vi "ModbusMaster.vi"(11 "queue in":refnum<queue>) -> ()   [LabVIEW 2014]
uses:
  controls/UI Data.ctl
  Project/Software/MyRIO Testing Software/Modbus.ctl
  <vilib>/Modbus/subvis/Modbus API/Modbus API.lvclass/Modbus API.ctl
  <vilib>/Modbus/subvis/Transmission Data Unit (ADU)/Transmission Data Unit/Transmission Data Unit.lvclass/Transmission Data Unit.ctl
  controls/Control ConfigurationSam.ctl
  <vilib>/Modbus/master/Modbus Master.lvclass
  <vilib>/Modbus/master/Data Access/Read Timeout/Set Read Timeout.vi
  <vilib>/Modbus/master/Data Access/Write Timeout/Set Write Timeout.vi
  <vilib>/Modbus/subvis/Modbus API/Read Transmission Data Unit.vi
  <vilib>/Modbus/subvis/Modbus API/Write Transmission Data Unit.vi
  <vilib>/Modbus/subvis/Transmission Data Unit (ADU)/Transmission Data Unit/Data Access/timeouts/Write read operation timeout.vi
  <vilib>/Modbus/subvis/Transmission Data Unit (ADU)/Transmission Data Unit/Data Access/timeouts/Write write operation timeout.vi
  <vilib>/Modbus/master/Data Access/Unit ID/Set Unit ID Property.vi
  <vilib>/Modbus/subvis/Transmission Data Unit (ADU)/Transmission Data Unit/Data Access/Unit ID/Write Unit ID.vi
  <vilib>/Modbus/master/Create Master Instance (Serial).vi
  <vilib>/Modbus/subvis/Transmission Data Unit (ADU)/Transmission Data Unit/Transmission Data Unit.lvclass
panel:
  out "PSoC PID Value":dbl
  out "Kp5":dbl=4.0
  out "Ki5":dbl=0.001
  out "Kd5":dbl
  in  "PIDScaler5":dbl=1000.0
  out "X":dbl
  out "Actual Values Written5":u16[](array[numeric])
  out "LabVIEW Heading":dbl
  out "Y":dbl
  out "PSoC Heading":dbl
  out "Values Read5":u16[](array[numeric])
  out "Values Read2":u16[](array[numeric])
  out "PositionLow2":u16
  out "PositionHigh2":i16
  out "SpeedRPS2":dbl
  out "SpeedRPM2":i16
  out "Motor Current2":dbl
  out "Position Full2":i32
  out "Setpoint Speed2":i16
  out "Actual Values Written2":u16[](array[numeric])
  out "Kd2":dbl
  out "Ki2":dbl=0.001
  out "Kp2":dbl=4.0
  in  "PIDScaler2":dbl=1000.0
  out "Values Read1":u16[](array[numeric])
  out "PositionLow1":u16
  out "PositionHigh1":i16
  out "SpeedRPS1":dbl
  out "SpeedRPM1":i16
  out "Motor Current1":dbl
  out "Position Full1":i32
  out "Setpoint Speed1":i16
  out "Actual Values Written1":u16[](array[numeric])
  out "Kd1":dbl
  out "Ki1":dbl=0.001
  out "Kp1":dbl=4.0
  in  "PIDScaler1":dbl=1000.0
  out "Setpoint Speed3":i16
  out "Actual Values Written3":u16[](array[numeric])
  out "Kd3":dbl
  out "Ki3":dbl=0.001
  out "Kp3":dbl=4.0
  in  "PIDScaler3":dbl=1000.0
  out "Values Read3":u16[](array[numeric])
  out "PositionLow3":u16
  out "PositionHigh3":i16
  out "SpeedRPS3":dbl
  out "SpeedRPM3":i16
  out "Motor Current3":dbl
  out "Position Full3":i32
  in  "PIDScaler4":dbl=1000.0
  out "Kp4":dbl=4.0
  out "Ki4":dbl=0.001
  out "Kd4":dbl
  out "Actual Values Written4":u16[](array[numeric])
  out "Setpoint Speed4":i16
  out "Position Full4":i32
  out "Motor Current4":dbl
  out "SpeedRPM4":i16
  out "SpeedRPS4":dbl
  out "PositionHigh4":i16
  out "PositionLow4":u16
  out "Values Read4":u16[](array[numeric])
  in  "Coil Values to Write":bool[](array[boolean])
  in  "Read Count 2":u16=10
  out "Coil Values Read":bool[](array[boolean])
  in  "flow control":u16(ring) items=["None", "XON/XOFF", "RTS/CTS", "XON/XOFF & RTS/CTS", "DTR/DSR", "XON/XOFF & DTR/DSR"]
  in  "parity":u16(ring) items=["None", "Odd", "Even"]
  in  "StartingSlave ID":u8=4
  in  "serial type":enum16{"RTU", "ASCII"}(ring)
  in  "VISA resource name":refnum<visa-resource-name>="ASRL3::INSTR"
  in  "baud rate":u32=115200
  # "Modbus Controller"
  # "Motor 1"
  # "Motor 2"
  # "Motor 3"
  # "Motor 4"
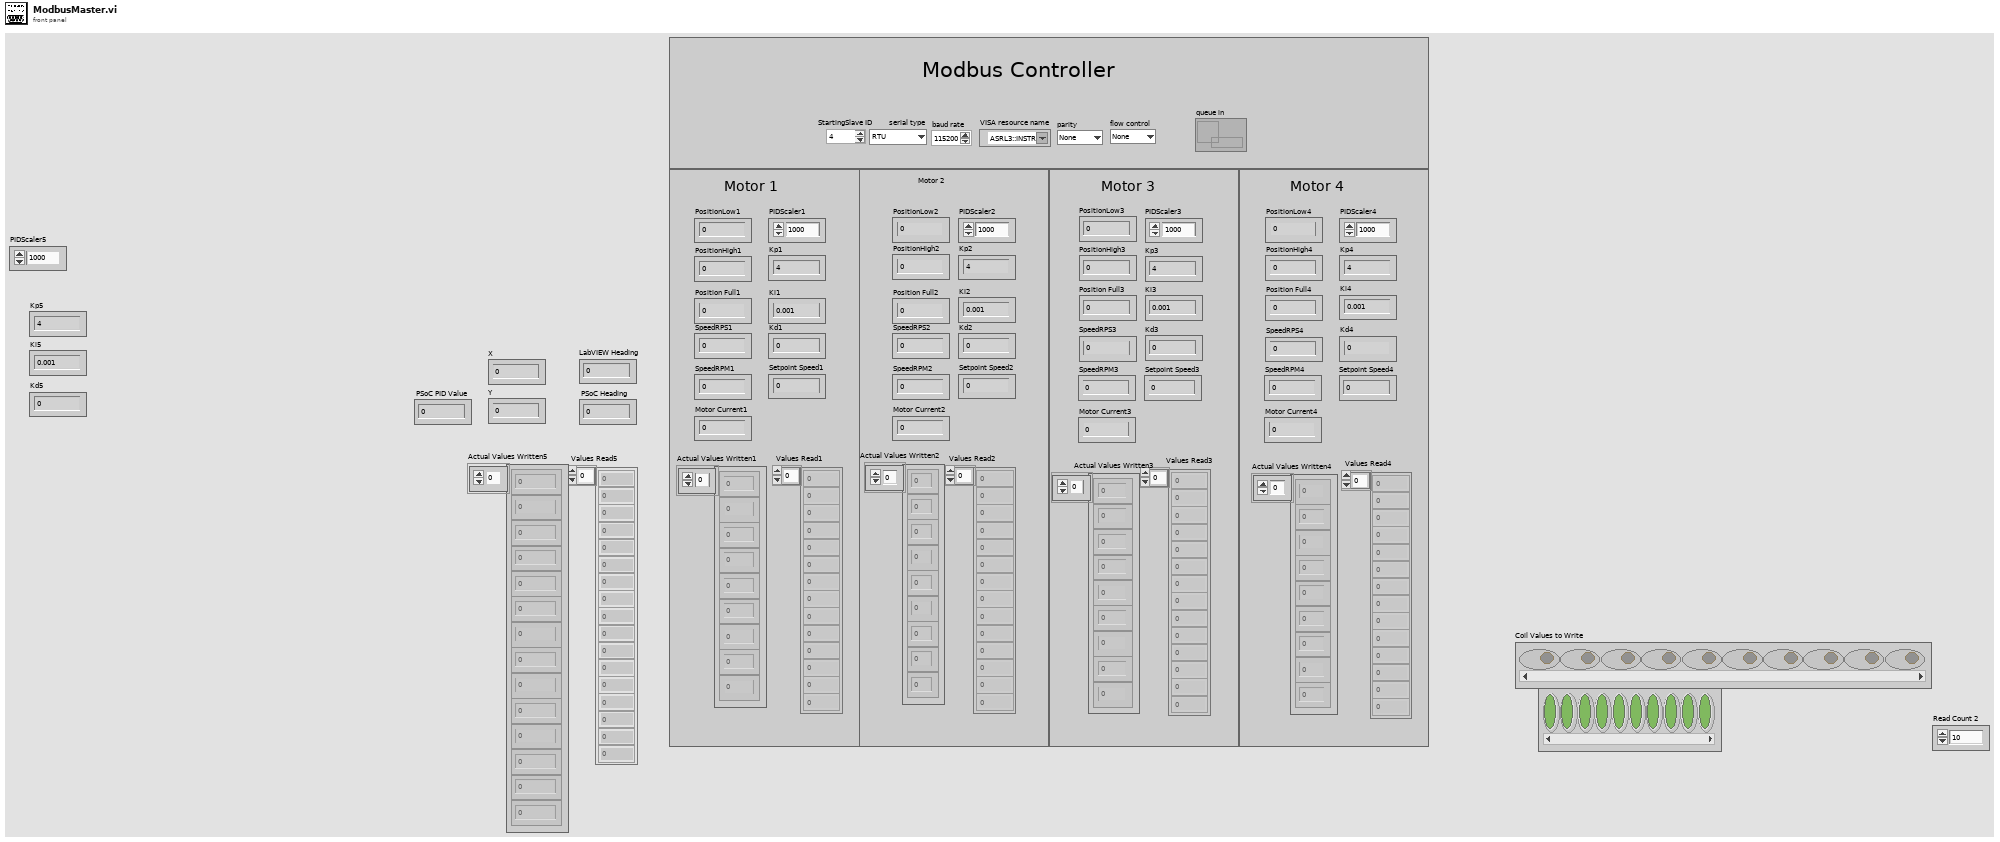
[diagram p1: front panel]
types:
  T1 = typedef "Modbus.ctl" = enum16{"Create Master", "Write Slave 1", "Write Slave 2", "Write Slave 3", "Write Slave 4", "Write Slave 5", "Read Slave 1", "Read Slave 2", "Read Slave 3", "Read Slave 4", "Read Slave 5", "Close Master", "TestReadCoils4", "TestWriteCoils4"}
  T2 = typedef "Control ConfigurationSam.ctl" = cluster{"PID Gains":cluster{"proportional gain (Kc)":dbl, "integral gain (Kc*Ts/Ti)":dbl, "derivative gain (Kc*Td/Ts)":dbl}}
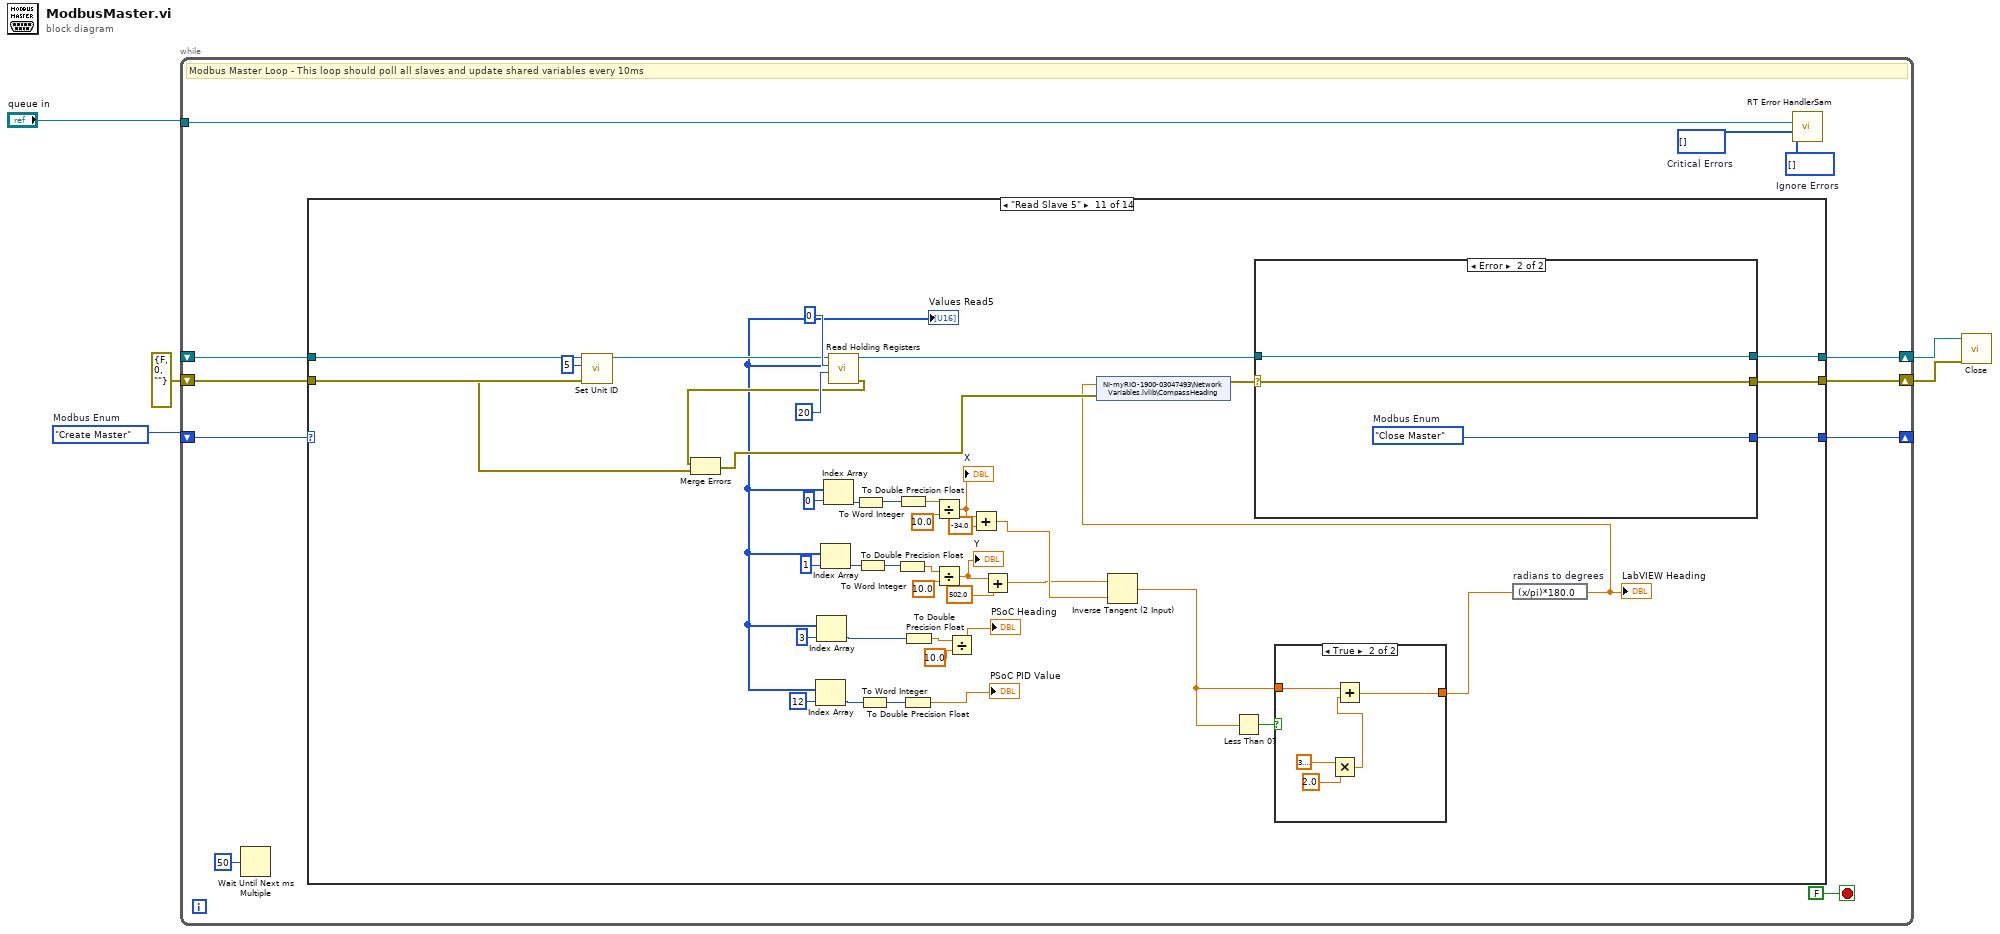
[diagram p0: block diagram]
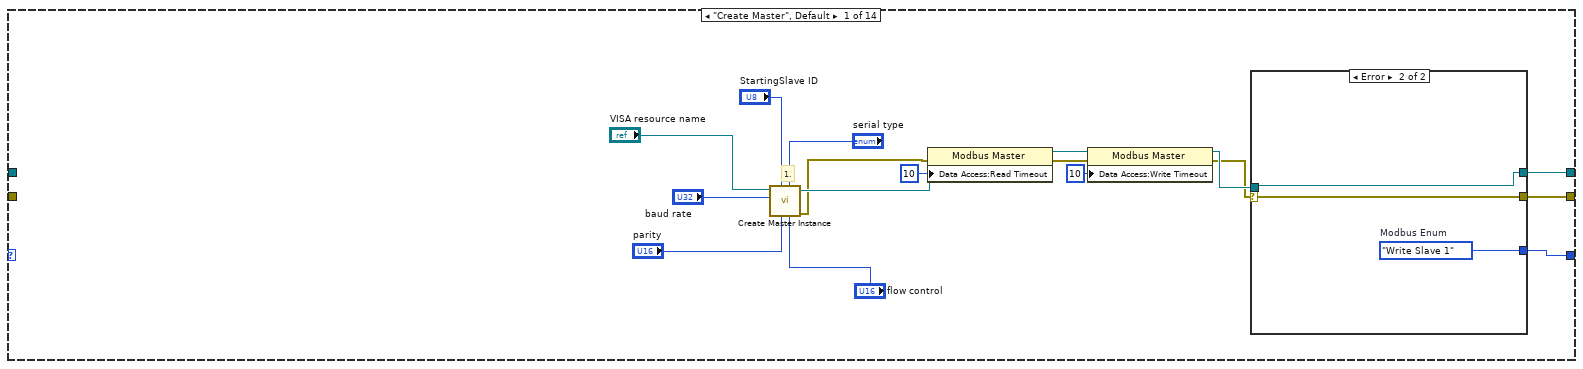
[diagram p2: hidden frame]
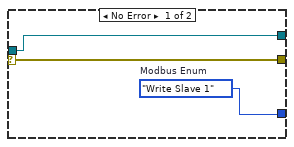
[diagram p3: hidden frame]
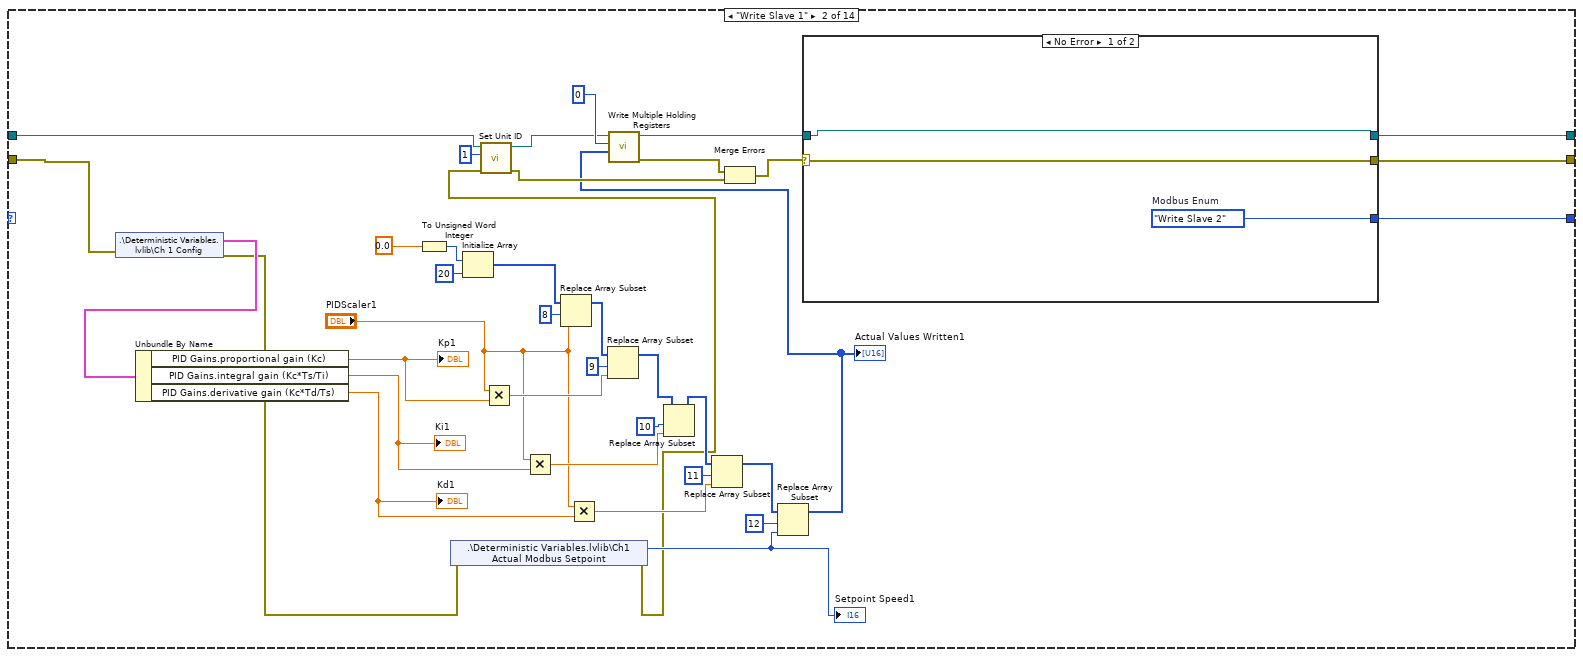
[diagram p4: hidden frame]
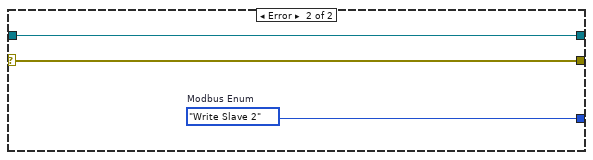
[diagram p5: hidden frame]
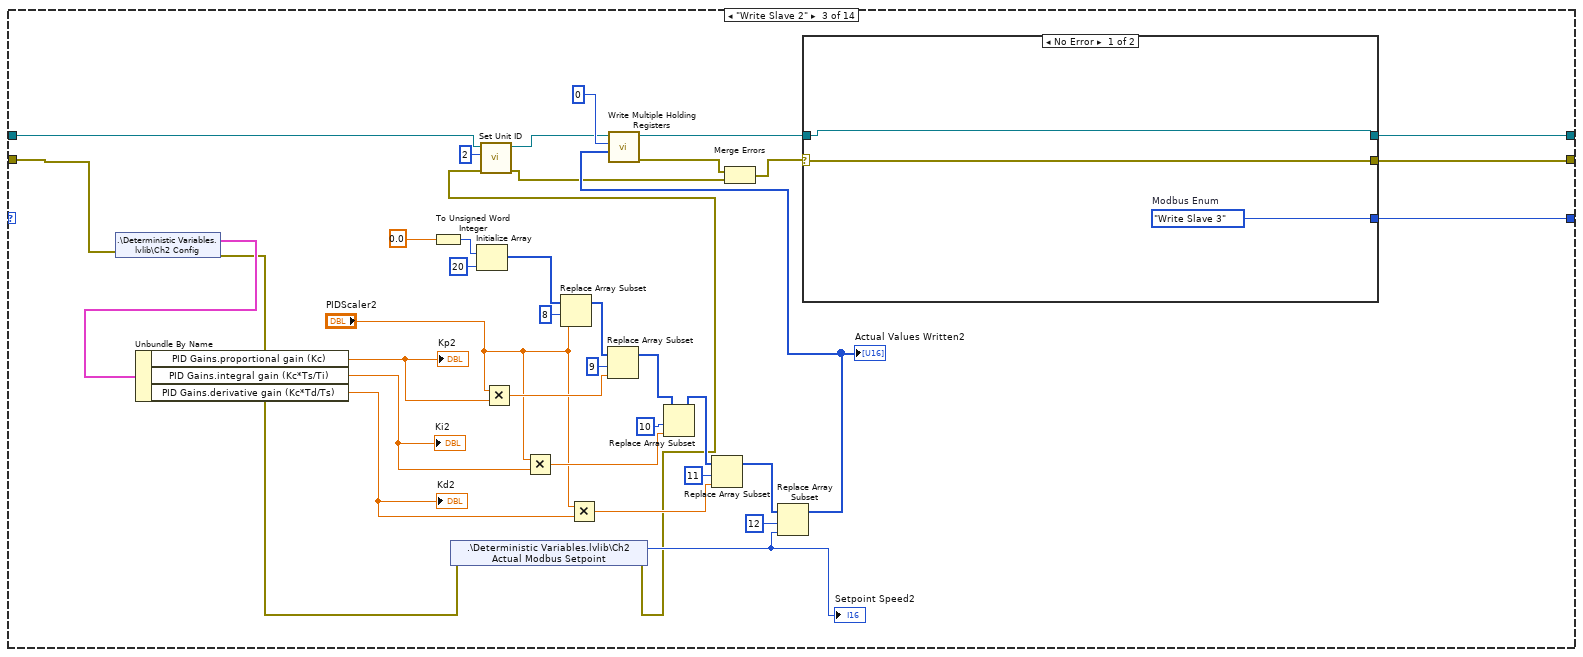
[diagram p6: hidden frame]
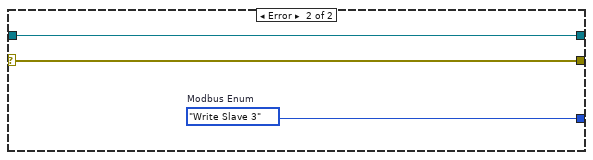
[diagram p7: hidden frame]
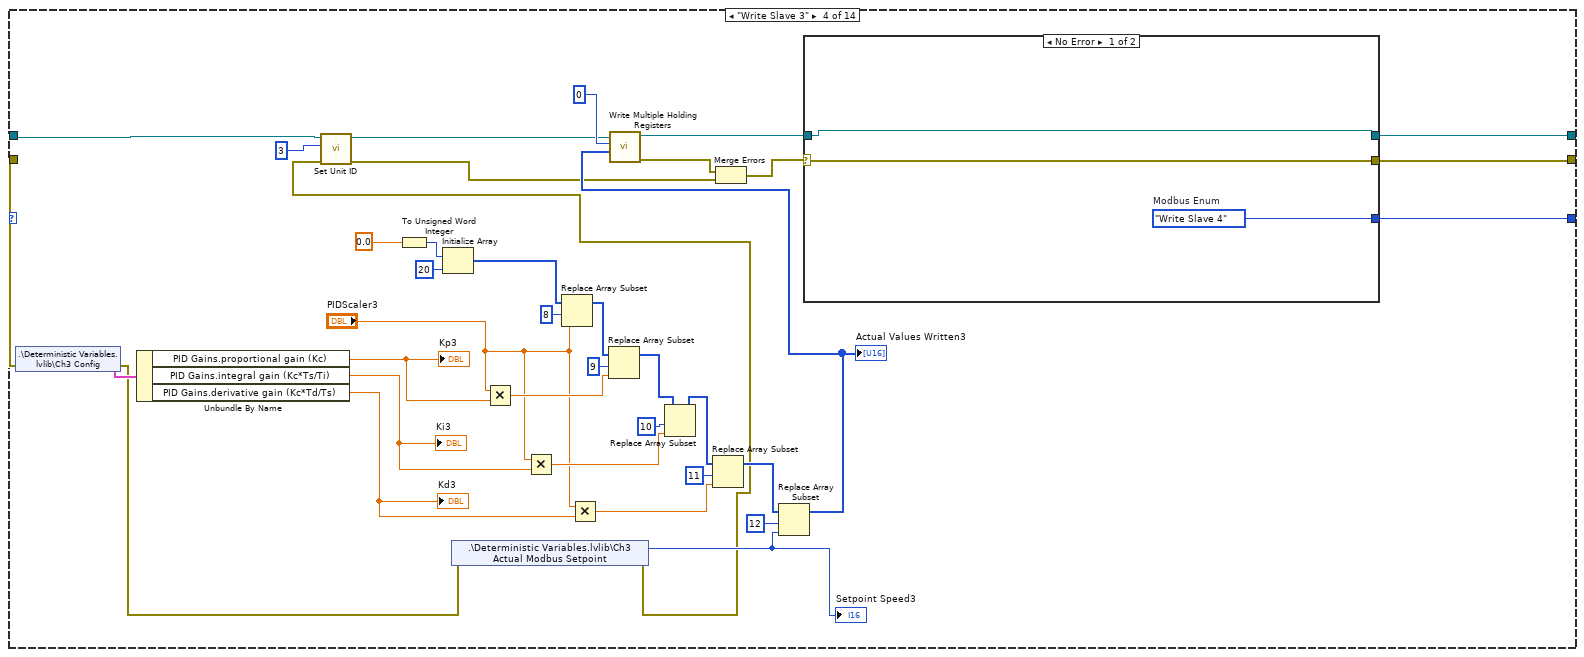
[diagram p8: hidden frame]
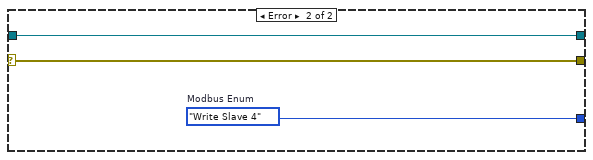
[diagram p9: hidden frame]
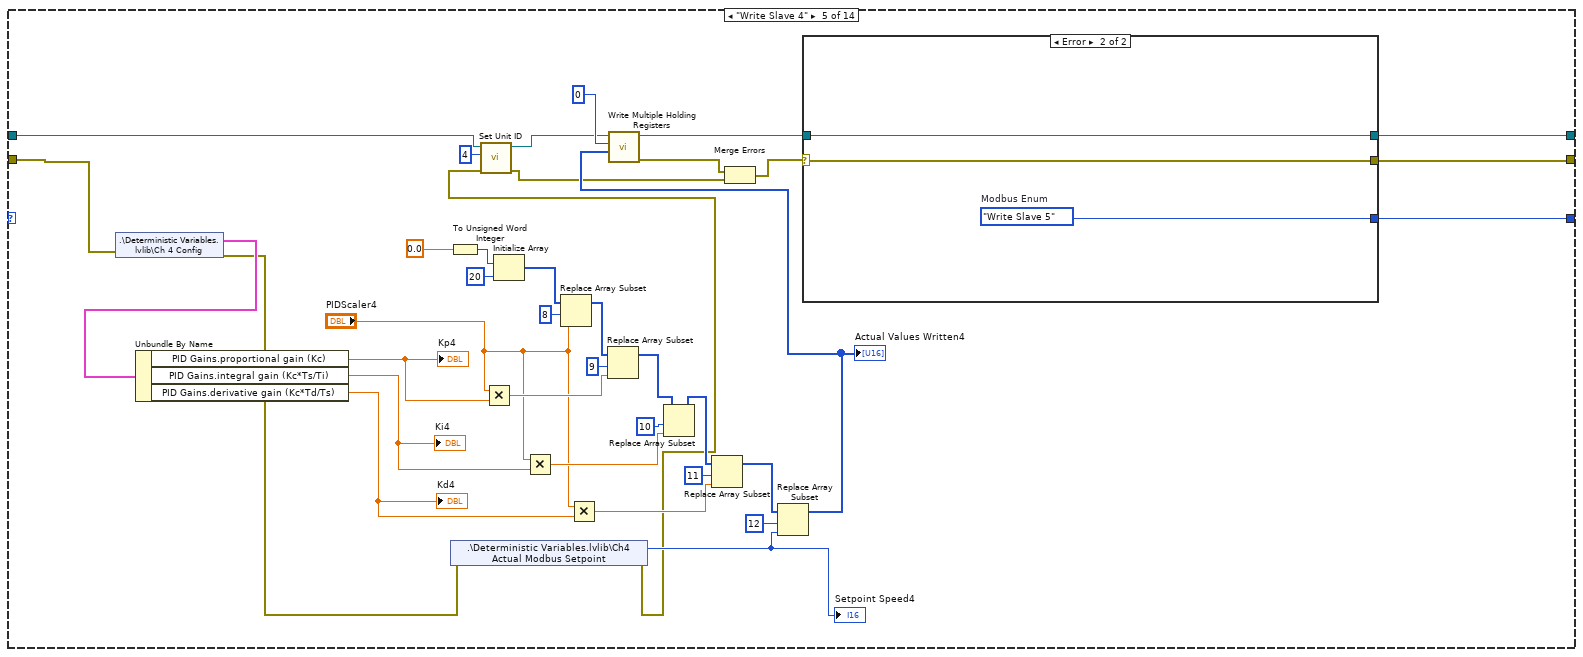
[diagram p10: hidden frame]
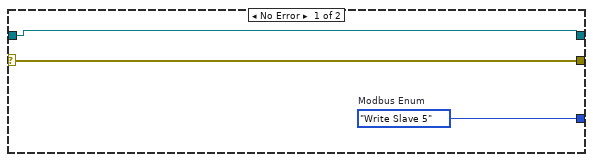
[diagram p11: hidden frame]
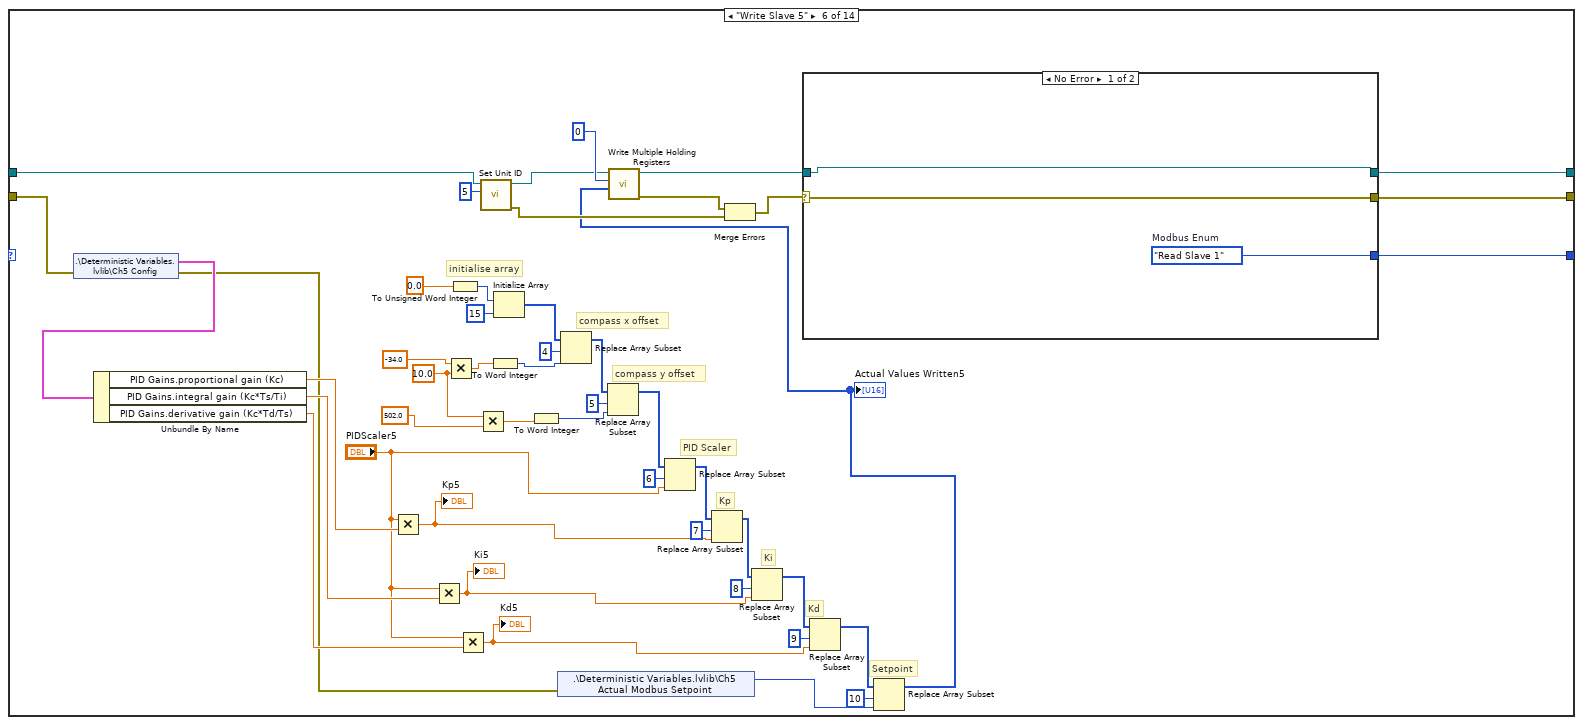
[diagram p12: hidden frame]
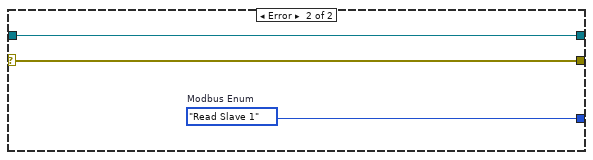
[diagram p13: hidden frame]
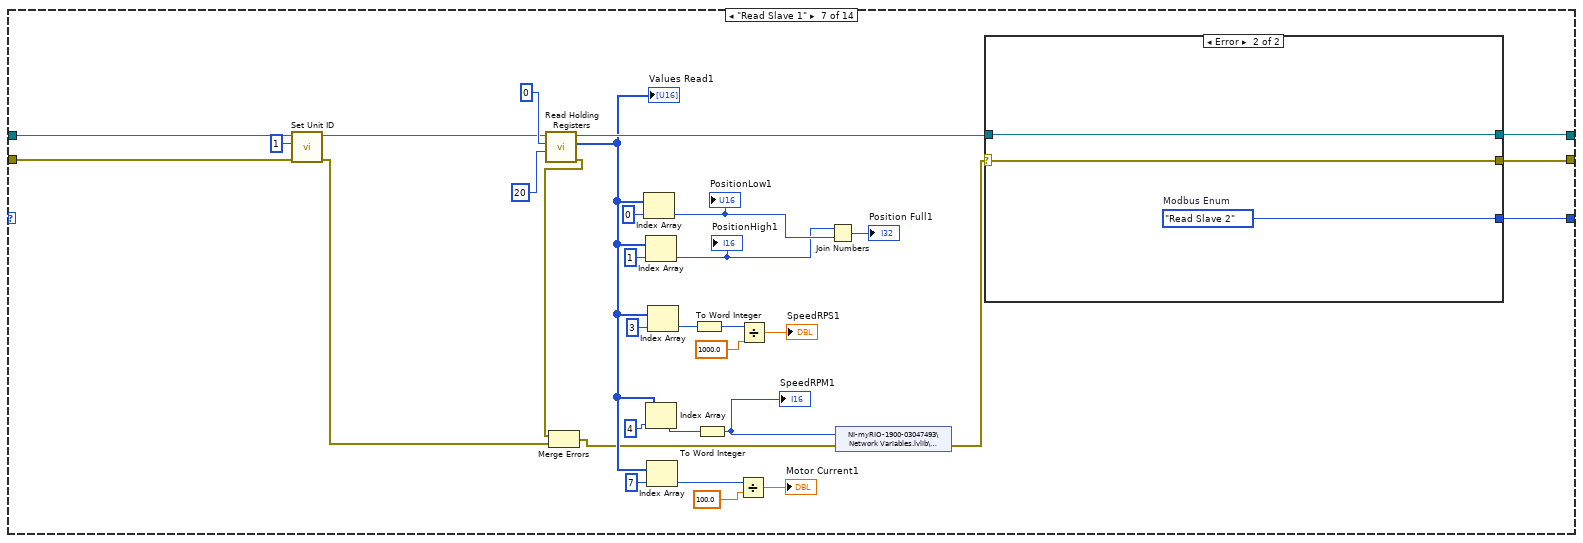
[diagram p14: hidden frame]
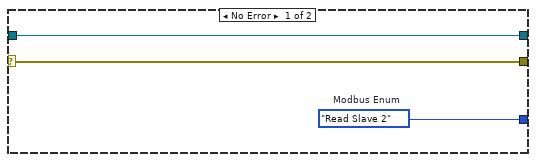
[diagram p15: hidden frame]
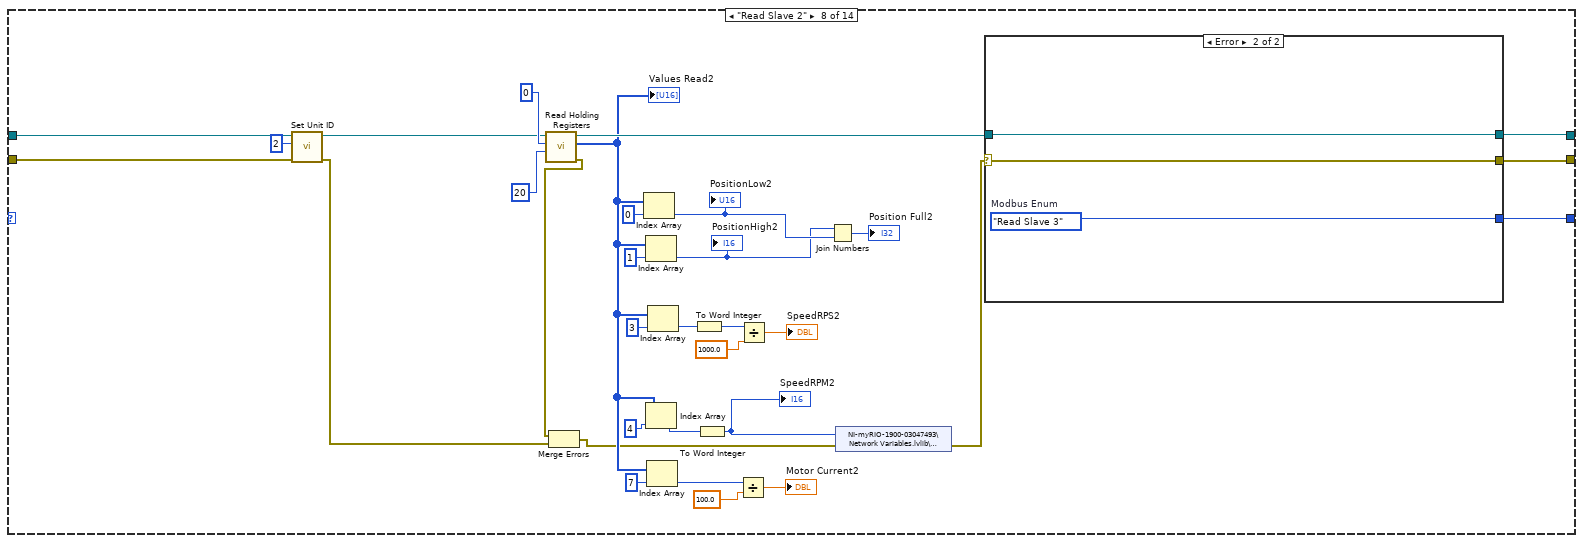
[diagram p16: hidden frame]
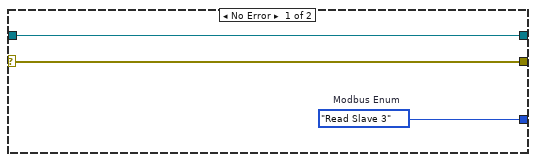
[diagram p17: hidden frame]
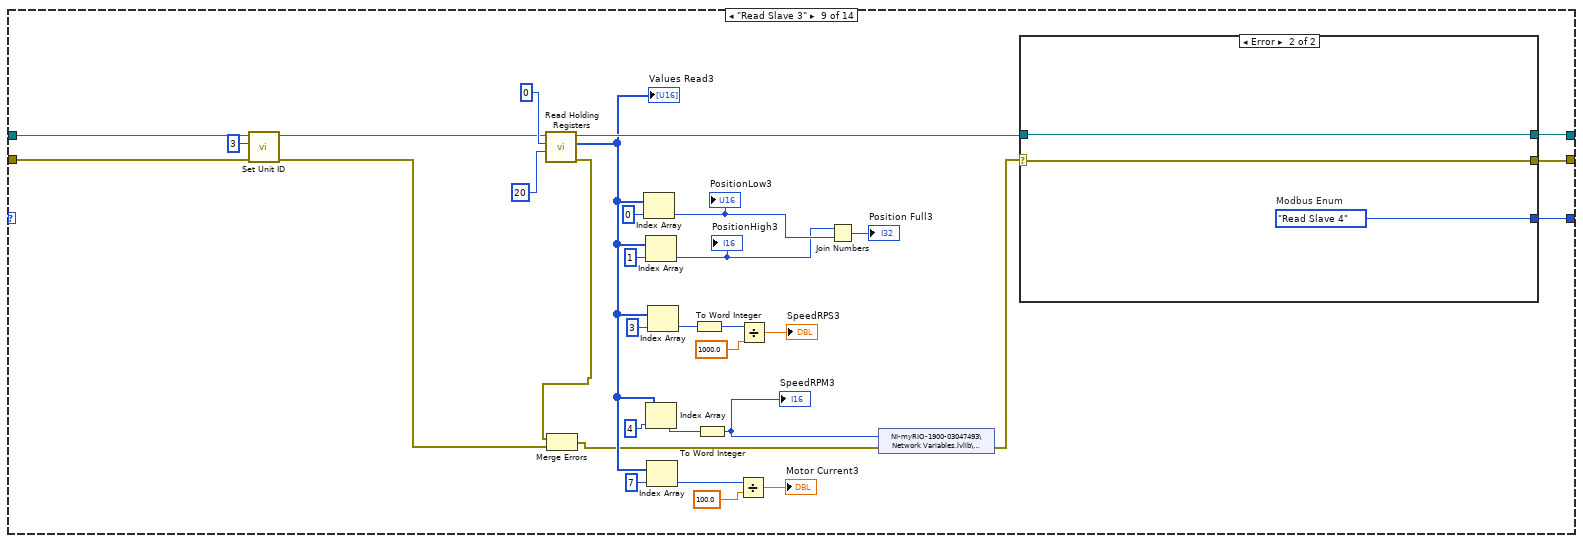
[diagram p18: hidden frame]
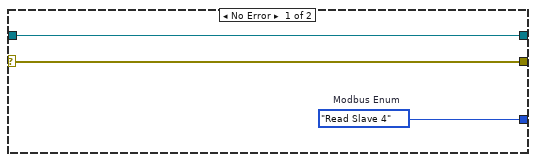
[diagram p19: hidden frame]
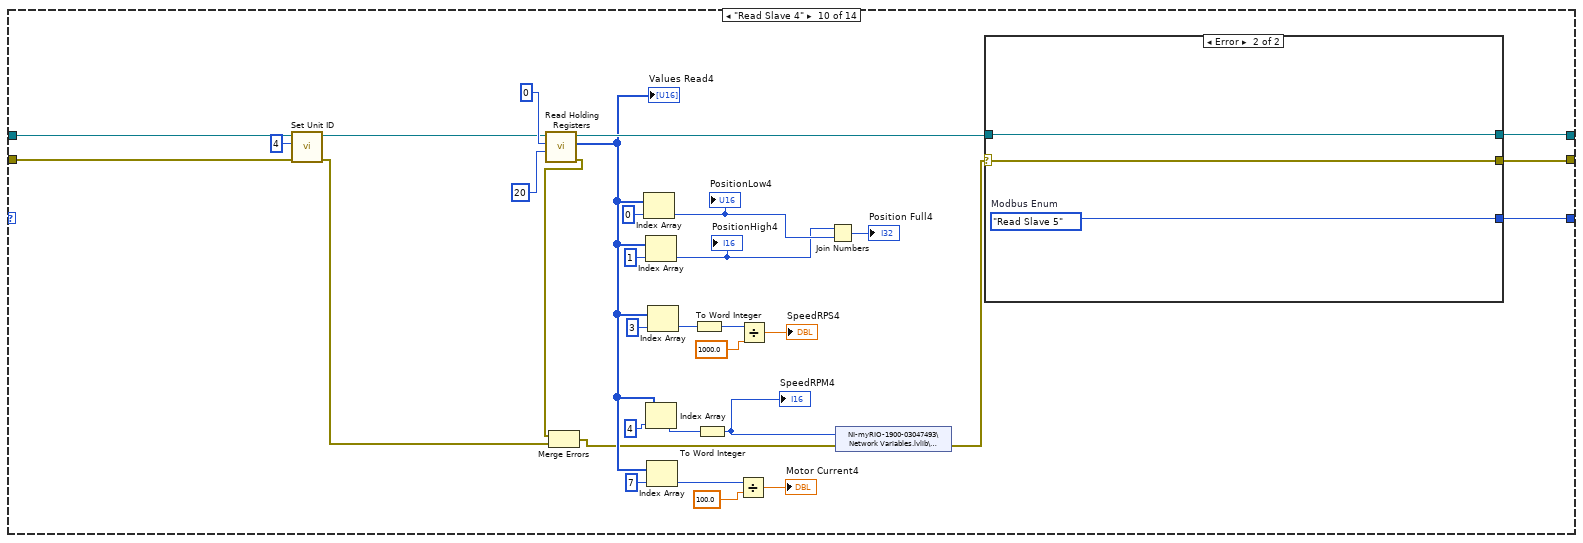
[diagram p20: hidden frame]
diagram:
  w2 = Modbus."Create Master"  # Modbus Enum
  n1 = while {
    tunnel: "queue in" -> [w13]
    shift-right: [w12] -> w4
    shift-left: _ -> [w10]
    shift-right: [w11] -> w3
    shift-left: errorcluster {"status"=FALSE, "code"=0, "source"=""} ("error IO") -> [w6]
    shift-right: [w7] -> _
    shift-left: w2 -> [w8]
    stop <- FALSE stop-if-true
    w14 = i32[] []  # Critical Errors
    w15 = i32[] []  # Ignore Errors
    # "Modbus Master Loop - This loop should poll all slaves and update shared variables every 10ms"
    n2 = Wait Until Next ms Multiple(millisecond multiple=u32 50) -> ()  [unwired: 1 out]
    n3 = case shown="\"Read Slave 5\"" w8 {
      tunnel: [w27 w75 w118 w161 w204 w257 w295 w333 w371 w409 w459 refnum<class "Modbus Master.lvclass"> refnum ("Modbus master out") w480 w495] -> w12
      tunnel: [w26 w74 w117 w160 w203 w256 w296 w334 w372 w410 w460 errorcluster {"status"=FALSE, "code"=0, "source"=""} ("error IO") w487 w494] -> w11
      tunnel: w10 -> [_ w50 w92 w134 w178 w251 w269 w307 w347 w383 w451 w477 w484 w500]
      tunnel: w6 -> [_ w57 w99 w142 w185 w232 w270 w308 w346 w384 w452 w476 w483 w499]
      tunnel: [w25 w76 w119 w162 w205 w258 w294 w332 w370 w408 w458 w473 w478 w496] -> w7
      frame "Create Master", Default {
        # "1."
        n4 = call-poly <vilib>:"Create Master Instance.vi"("flow control (None)"="flow control", "serial type"="serial type", "parity (Even)"="parity", "unit ID"="StartingSlave ID", "baud rate (9600)"="baud rate", "VISA resource name"="VISA resource name") -> ("error out"=w22:errorcluster, "serial master instance"=w24:refnum<class "Modbus Master.lvclass">)  [unwired: 4 in]
        n5 = property class="Modbus Master"(reference=w24, error in=w22, "Data Access:Read Timeout"=10 ("Read Timeout")) -> (reference out=w21:refnum<class "Modbus Master.lvclass">, error out=w20:errorcluster)
        n6 = property class="Modbus Master"(reference=w21, error in=w20, "Data Access:Write Timeout"=10 ("Write Timeout")) -> (reference out=w18:refnum<class "Modbus Master.lvclass">, error out=w17:errorcluster)
        n7 = case shown="Error" w17 {
          selector: w17 -> [w35 w39]
          tunnel: w18 -> [w36 w38]
          tunnel: [w36 w38] -> w27
          tunnel: [w35 w39] -> w26
          tunnel: [w34 w37] -> w25
          frame No Error {
            w34 = Modbus."Write Slave 1"  # Modbus Enum
          }
          frame Error {
            w37 = Modbus."Write Slave 1"  # Modbus Enum
          }
        }
      }
      frame "Write Slave 1" {
        n8 = shared-variable ".\\Deterministic Variables.lvlib\\Ch 1 Config"(error in=w57) -> (w56:T2, error out=w52:errorcluster)
        n9 = Unbundle By Name(w56) -> ("PID Gains.proportional gain (Kc)"=w55:dbl, "PID Gains.integral gain (Kc*Ts/Ti)"=w54:dbl, "PID Gains.derivative gain (Kc*Td/Ts)"=w53:dbl)
        "Kd1" <- w53
        "Ki1" <- w54
        "Kp1" <- w55
        n10 = To Unsigned Word Integer(number=0.0 ("element")) -> (unsigned 16bit integer=w41:u16)
        n11 = shared-variable ".\\Deterministic Variables.lvlib\\Ch1 Actual Modbus Setpoint"(error in=w52) -> (w58:i16, error out=w51:errorcluster)
        "Setpoint Speed1" <- w58
        n12 = Initialize Array(w41, 20 ("dimension size")) -> (w40:u16[])
        n13 = call <vilib>:"Set Unit ID.vi"("error in (no error)"=w51, "unit ID"=u8 1, "Modbus master in"=w50) -> ("error out"=w45:errorcluster, "Modbus master out"=w49:refnum<class "Modbus Master.lvclass">)  [unwired: 7 in]
        n14 = Multiply(x="PIDScaler1", y=w55) -> (x*y=w65:dbl)
        n15 = Multiply(x="PIDScaler1", y=w54) -> (x*y=w64:dbl)
        n16 = Replace Array Subset(array=w40, new element="PIDScaler1", index=8) -> (w66:u16[])
        n17 = Multiply(x="PIDScaler1", y=w53) -> (x*y=w62:dbl)
        n18 = Replace Array Subset(array=w66, new element=w65, index=9) -> (w61:u16[])
        n19 = Replace Array Subset(array=w61, new element=w64, index=10) -> (w60:u16[])
        n20 = Replace Array Subset(array=w60, new element=w62, index=11) -> (w59:u16[])
        n21 = Replace Array Subset(array=w59, new element=w58, index=12) -> (w44:u16[])
        "Actual Values Written1" <- w44
        n22 = call-dynamic "Write Multiple Holding Registers.vi"("holding register values"=w44, "starting address"=u16 0, "Modbus master in"=w49) -> ("error out"=w47:errorcluster, "Modbus master out"=w72:refnum<class "Modbus Master.lvclass">)  [unwired: 7 in]
        n23 = Merge Errors(w47, w45) -> (w46:errorcluster)
        n24 = case shown="No Error" w46 {
          selector: w46 -> [w78 w81]
          tunnel: w72 -> [w79 w82]
          tunnel: [w77 w80] -> w76
          tunnel: [w79 w82] -> w75
          tunnel: [w78 w81] -> w74
          frame No Error {
            w77 = Modbus."Write Slave 2"  # Modbus Enum
          }
          frame Error {
            w80 = Modbus."Write Slave 2"  # Modbus Enum
          }
        }
      }
      frame "Write Slave 2" {
        n25 = shared-variable ".\\Deterministic Variables.lvlib\\Ch2 Config"(error in=w99) -> (w98:T2, error out=w94:errorcluster)
        n26 = Unbundle By Name(w98) -> ("PID Gains.proportional gain (Kc)"=w97:dbl, "PID Gains.integral gain (Kc*Ts/Ti)"=w96:dbl, "PID Gains.derivative gain (Kc*Td/Ts)"=w95:dbl)
        "Kd2" <- w95
        "Ki2" <- w96
        "Kp2" <- w97
        n27 = To Unsigned Word Integer(number=0.0 ("element")) -> (unsigned 16bit integer=w84:u16)
        n28 = shared-variable ".\\Deterministic Variables.lvlib\\Ch2 Actual Modbus Setpoint"(error in=w94) -> (w100:i16, error out=w93:errorcluster)
        "Setpoint Speed2" <- w100
        n29 = Initialize Array(w84, 20 ("dimension size")) -> (w83:u16[])
        n30 = call <vilib>:"Set Unit ID.vi"("error in (no error)"=w93, "unit ID"=u8 2, "Modbus master in"=w92) -> ("error out"=w87:errorcluster, "Modbus master out"=w91:refnum<class "Modbus Master.lvclass">)  [unwired: 7 in]
        n31 = Multiply(x="PIDScaler2", y=w97) -> (x*y=w108:dbl)
        n32 = Multiply(x="PIDScaler2", y=w96) -> (x*y=w107:dbl)
        n33 = Replace Array Subset(array=w83, new element="PIDScaler2", index=8) -> (w109:u16[])
        n34 = Multiply(x="PIDScaler2", y=w95) -> (x*y=w105:dbl)
        n35 = Replace Array Subset(array=w109, new element=w108, index=9) -> (w104:u16[])
        n36 = Replace Array Subset(array=w104, new element=w107, index=10) -> (w103:u16[])
        n37 = Replace Array Subset(array=w103, new element=w105, index=11) -> (w102:u16[])
        n38 = Replace Array Subset(array=w102, new element=w100, index=12) -> (w101:u16[])
        "Actual Values Written2" <- w101
        n39 = call-dynamic "Write Multiple Holding Registers.vi"("holding register values"=w101, "starting address"=u16 0, "Modbus master in"=w91) -> ("error out"=w89:errorcluster, "Modbus master out"=w115:refnum<class "Modbus Master.lvclass">)  [unwired: 7 in]
        n40 = Merge Errors(w89, w87) -> (w88:errorcluster)
        n41 = case shown="No Error" w88 {
          selector: w88 -> [w121 w124]
          tunnel: w115 -> [w122 w125]
          tunnel: [w120 w123] -> w119
          tunnel: [w122 w125] -> w118
          tunnel: [w121 w124] -> w117
          frame No Error {
            w120 = Modbus."Write Slave 3"  # Modbus Enum
          }
          frame Error {
            w123 = Modbus."Write Slave 3"  # Modbus Enum
          }
        }
      }
      frame "Write Slave 3" {
        n42 = shared-variable ".\\Deterministic Variables.lvlib\\Ch3 Config"(error in=w142) -> (w141:T2, error out=w137:errorcluster)
        n43 = Unbundle By Name(w141) -> ("PID Gains.proportional gain (Kc)"=w140:dbl, "PID Gains.integral gain (Kc*Ts/Ti)"=w139:dbl, "PID Gains.derivative gain (Kc*Td/Ts)"=w138:dbl)
        "Kd3" <- w138
        "Ki3" <- w139
        "Kp3" <- w140
        n44 = To Unsigned Word Integer(number=0.0 ("element")) -> (unsigned 16bit integer=w127:u16)
        n45 = Initialize Array(w127, 20 ("dimension size")) -> (w126:u16[])
        n46 = shared-variable ".\\Deterministic Variables.lvlib\\Ch3 Actual Modbus Setpoint"(error in=w137) -> (w143:i16, error out=w133:errorcluster)
        "Setpoint Speed3" <- w143
        n47 = call <vilib>:"Set Unit ID.vi"("error in (no error)"=w133, "unit ID"=u8 3, "Modbus master in"=w134) -> ("error out"=w130:errorcluster, "Modbus master out"=w136:refnum<class "Modbus Master.lvclass">)  [unwired: 7 in]
        n48 = Multiply(x="PIDScaler3", y=w140) -> (x*y=w151:dbl)
        n49 = Multiply(x="PIDScaler3", y=w139) -> (x*y=w150:dbl)
        n50 = Replace Array Subset(array=w126, new element="PIDScaler3", index=8) -> (w152:u16[])
        n51 = Multiply(x="PIDScaler3", y=w138) -> (x*y=w148:dbl)
        n52 = Replace Array Subset(array=w152, new element=w151, index=9) -> (w147:u16[])
        n53 = Replace Array Subset(array=w147, new element=w150, index=10) -> (w146:u16[])
        n54 = Replace Array Subset(array=w146, new element=w148, index=11) -> (w145:u16[])
        n55 = Replace Array Subset(array=w145, new element=w143, index=12) -> (w144:u16[])
        "Actual Values Written3" <- w144
        n56 = call-dynamic "Write Multiple Holding Registers.vi"("holding register values"=w144, "starting address"=u16 0, "Modbus master in"=w136) -> ("error out"=w131:errorcluster, "Modbus master out"=w158:refnum<class "Modbus Master.lvclass">)  [unwired: 7 in]
        n57 = Merge Errors(w131, w130) -> (w132:errorcluster)
        n58 = case shown="No Error" w132 {
          selector: w132 -> [w164 w167]
          tunnel: w158 -> [w165 w168]
          tunnel: [w163 w166] -> w162
          tunnel: [w165 w168] -> w161
          tunnel: [w164 w167] -> w160
          frame No Error {
            w163 = Modbus."Write Slave 4"  # Modbus Enum
          }
          frame Error {
            w166 = Modbus."Write Slave 4"  # Modbus Enum
          }
        }
      }
      frame "Write Slave 4" {
        n59 = shared-variable ".\\Deterministic Variables.lvlib\\Ch 4 Config"(error in=w185) -> (w184:T2, error out=w180:errorcluster)
        n60 = Unbundle By Name(w184) -> ("PID Gains.proportional gain (Kc)"=w183:dbl, "PID Gains.integral gain (Kc*Ts/Ti)"=w182:dbl, "PID Gains.derivative gain (Kc*Td/Ts)"=w181:dbl)
        "Kd4" <- w181
        "Ki4" <- w182
        "Kp4" <- w183
        n61 = To Unsigned Word Integer(number=0.0 ("element")) -> (unsigned 16bit integer=w170:u16)
        n62 = shared-variable ".\\Deterministic Variables.lvlib\\Ch4 Actual Modbus Setpoint"(error in=w180) -> (w186:i16, error out=w179:errorcluster)
        "Setpoint Speed4" <- w186
        n63 = call <vilib>:"Set Unit ID.vi"("error in (no error)"=w179, "unit ID"=u8 4, "Modbus master in"=w178) -> ("error out"=w173:errorcluster, "Modbus master out"=w177:refnum<class "Modbus Master.lvclass">)  [unwired: 7 in]
        n64 = Multiply(x="PIDScaler4", y=w183) -> (x*y=w194:dbl)
        n65 = Initialize Array(w170, 20 ("dimension size")) -> (w169:u16[])
        n66 = Multiply(x="PIDScaler4", y=w182) -> (x*y=w193:dbl)
        n67 = Replace Array Subset(array=w169, new element="PIDScaler4", index=8) -> (w195:u16[])
        n68 = Multiply(x="PIDScaler4", y=w181) -> (x*y=w191:dbl)
        n69 = Replace Array Subset(array=w195, new element=w194, index=9) -> (w190:u16[])
        n70 = Replace Array Subset(array=w190, new element=w193, index=10) -> (w189:u16[])
        n71 = Replace Array Subset(array=w189, new element=w191, index=11) -> (w188:u16[])
        n72 = Replace Array Subset(array=w188, new element=w186, index=12) -> (w187:u16[])
        "Actual Values Written4" <- w187
        n73 = call-dynamic "Write Multiple Holding Registers.vi"("holding register values"=w187, "starting address"=u16 0, "Modbus master in"=w177) -> ("error out"=w175:errorcluster, "Modbus master out"=w201:refnum<class "Modbus Master.lvclass">)  [unwired: 7 in]
        n74 = Merge Errors(w175, w173) -> (w174:errorcluster)
        n75 = case shown="Error" w174 {
          selector: w174 -> [w207 w210]
          tunnel: w201 -> [w208 w211]
          tunnel: [w206 w209] -> w205
          tunnel: [w208 w211] -> w204
          tunnel: [w207 w210] -> w203
          frame No Error {
            w206 = Modbus."Write Slave 5"  # Modbus Enum
          }
          frame Error {
            w209 = Modbus."Write Slave 5"  # Modbus Enum
          }
        }
      }
      frame "Write Slave 5" {
        w234 = 10.0 ("y")
        # "Setpoint"
        # "Kd"
        # "Ki"
        # "Kp"
        # "PID Scaler"
        # "compass y offset"
        # "compass x offset"
        # "initialise array"
        n76 = shared-variable ".\\Deterministic Variables.lvlib\\Ch5 Config"(error in=w232) -> (w233:T2, error out=w212:errorcluster)
        n77 = Unbundle By Name(w233) -> ("PID Gains.proportional gain (Kc)"=w223:dbl, "PID Gains.integral gain (Kc*Ts/Ti)"=w222:dbl, "PID Gains.derivative gain (Kc*Td/Ts)"=w221:dbl)
        n78 = Multiply(x="PIDScaler5", y=w223) -> (x*y=w219:dbl)
        "Kp5" <- w219
        n79 = Multiply(x="PIDScaler5", y=w222) -> (x*y=w218:dbl)
        "Ki5" <- w218
        n80 = Multiply(x=-34.0, y=w234) -> (x*y=w238:dbl)
        n81 = To Unsigned Word Integer(number=0.0 ("element")) -> (unsigned 16bit integer=w243:u16)
        n82 = Multiply(x="PIDScaler5", y=w221) -> (x*y=w217:dbl)
        "Kd5" <- w217
        n83 = Multiply(x=w234, y=502.0) -> (x*y=w236:dbl)
        n84 = call <vilib>:"Set Unit ID.vi"("unit ID"=u8 5, "Modbus master in"=w251) -> ("error out"=w246:errorcluster, "Modbus master out"=w250:refnum<class "Modbus Master.lvclass">)  [unwired: 8 in]
        n85 = To Word Integer(number=w238) -> (16bit integer=w240:i16)
        n86 = Initialize Array(w243, 15 ("dimension size")) -> (w242:u16[])
        n87 = To Word Integer(number=w236) -> (16bit integer=w239:i16)
        n88 = shared-variable ".\\Deterministic Variables.lvlib\\Ch5 Actual Modbus Setpoint"(error in=w212) -> (w213:i16)  [unwired: 1 out]
        n89 = Replace Array Subset(array=w242, new element=w240, index=4) -> (w252:u16[])
        n90 = Replace Array Subset(array=w252, new element=w239, index=5) -> (w228:u16[])
        n91 = Replace Array Subset(array=w228, new element="PIDScaler5", index=6) -> (w230:u16[])
        n92 = Replace Array Subset(array=w230, new element=w219, index=7) -> (w227:u16[])
        n93 = Replace Array Subset(array=w227, new element=w218, index=8) -> (w225:u16[])
        n94 = Replace Array Subset(array=w225, new element=w217, index=9) -> (w215:u16[])
        n95 = Replace Array Subset(array=w215, new element=w213, index=10) -> (w214:u16[])
        "Actual Values Written5" <- w214
        n96 = call-dynamic "Write Multiple Holding Registers.vi"("holding register values"=w214, "starting address"=u16 0, "Modbus master in"=w250) -> ("error out"=w248:errorcluster, "Modbus master out"=w254:refnum<class "Modbus Master.lvclass">)  [unwired: 7 in]
        n97 = Merge Errors(w248, w246) -> (w247:errorcluster)
        n98 = case shown="No Error" w247 {
          selector: w247 -> [w260 w263]
          tunnel: w254 -> [w261 w264]
          tunnel: [w259 w262] -> w258
          tunnel: [w261 w264] -> w257
          tunnel: [w260 w263] -> w256
          frame No Error {
            w259 = Modbus."Read Slave 1"  # Modbus Enum
          }
          frame Error {
            w262 = Modbus."Read Slave 1"  # Modbus Enum
          }
        }
      }
      frame "Read Slave 1" {
        n99 = call <vilib>:"Set Unit ID.vi"("error in (no error)"=w270, "unit ID"=u8 1, "Modbus master in"=w269) -> ("error out"=w265:errorcluster, "Modbus master out"=w271:refnum<class "Modbus Master.lvclass">)  [unwired: 7 in]
        n100 = call-dynamic "Read Holding Registers.vi"("number of holding registers"=u16 20, "starting address"=u16 0, "Modbus master in"=w271) -> ("error out"=w266:errorcluster, "register values"=w280:u16[], "Modbus master out"=w291:refnum<class "Modbus Master.lvclass">)  [unwired: 6 in]
        "Values Read1" <- w280
        n101 = Merge Errors(w266, w265) -> (w267:errorcluster)
        n102 = Index Array(array=w280, index=0) -> (element=w279:u16)
        "PositionLow1" <- w279
        n103 = Index Array(array=w280, index=1) -> (element=w278:u16)
        "PositionHigh1" <- w278
        n104 = Index Array(array=w280, index=4) -> (element=w274:u16)
        n105 = Index Array(array=w280, index=7) -> (element=w283:u16)
        n106 = Index Array(array=w280, index=3) -> (element=w276:u16)
        n107 = To Word Integer(number=w276) -> (16bit integer=w275:i16)
        n108 = To Word Integer(number=w274) -> (16bit integer=w273:i16)
        "SpeedRPM1" <- w273
        n109 = Divide(x=w283, y=100.0) -> (x/y=→"Motor Current1":dbl)
        n110 = Divide(x=w275, y=1000.0) -> (x/y=→"SpeedRPS1":dbl)
        n111 = Join Numbers(hi=w278, lo=w279) -> ((hi.lo)=→"Position Full1":u32)
        n112 = shared-variable "NI-myRIO-1900-03047493\\Network Variables.lvlib\\SpeedMotor1"(w273, error in=w267) -> (error out=w272:errorcluster)
        n113 = case shown="Error" w272 {
          selector: w272 -> [w299 w302]
          tunnel: [w297 w300] -> w294
          tunnel: [w299 w302] -> w296
          tunnel: w291 -> [w298 w301]
          tunnel: [w298 w301] -> w295
          frame No Error {
            w297 = Modbus."Read Slave 2"  # Modbus Enum
          }
          frame Error {
            w300 = Modbus."Read Slave 2"  # Modbus Enum
          }
        }
      }
      frame "Read Slave 2" {
        n114 = call <vilib>:"Set Unit ID.vi"("error in (no error)"=w308, "unit ID"=u8 2, "Modbus master in"=w307) -> ("error out"=w303:errorcluster, "Modbus master out"=w309:refnum<class "Modbus Master.lvclass">)  [unwired: 7 in]
        n115 = call-dynamic "Read Holding Registers.vi"("number of holding registers"=u16 20, "starting address"=u16 0, "Modbus master in"=w309) -> ("error out"=w304:errorcluster, "register values"=w318:u16[], "Modbus master out"=w329:refnum<class "Modbus Master.lvclass">)  [unwired: 6 in]
        "Values Read2" <- w318
        n116 = Merge Errors(w304, w303) -> (w305:errorcluster)
        n117 = Index Array(array=w318, index=0) -> (element=w317:u16)
        "PositionLow2" <- w317
        n118 = Index Array(array=w318, index=1) -> (element=w316:u16)
        "PositionHigh2" <- w316
        n119 = Index Array(array=w318, index=4) -> (element=w312:u16)
        n120 = Index Array(array=w318, index=7) -> (element=w321:u16)
        n121 = Index Array(array=w318, index=3) -> (element=w314:u16)
        n122 = To Word Integer(number=w314) -> (16bit integer=w313:i16)
        n123 = To Word Integer(number=w312) -> (16bit integer=w311:i16)
        "SpeedRPM2" <- w311
        n124 = Divide(x=w321, y=100.0) -> (x/y=→"Motor Current2":dbl)
        n125 = Divide(x=w313, y=1000.0) -> (x/y=→"SpeedRPS2":dbl)
        n126 = Join Numbers(hi=w316, lo=w317) -> ((hi.lo)=→"Position Full2":u32)
        n127 = shared-variable "NI-myRIO-1900-03047493\\Network Variables.lvlib\\SpeedMotor2"(w311, error in=w305) -> (error out=w310:errorcluster)
        n128 = case shown="Error" w310 {
          selector: w310 -> [w337 w340]
          tunnel: [w335 w338] -> w332
          tunnel: [w337 w340] -> w334
          tunnel: w329 -> [w336 w339]
          tunnel: [w336 w339] -> w333
          frame No Error {
            w335 = Modbus."Read Slave 3"  # Modbus Enum
          }
          frame Error {
            w338 = Modbus."Read Slave 3"  # Modbus Enum
          }
        }
      }
      frame "Read Slave 3" {
        n129 = call <vilib>:"Set Unit ID.vi"("error in (no error)"=w346, "unit ID"=u8 3, "Modbus master in"=w347) -> ("error out"=w341:errorcluster, "Modbus master out"=w344:refnum<class "Modbus Master.lvclass">)  [unwired: 7 in]
        n130 = call-dynamic "Read Holding Registers.vi"("number of holding registers"=u16 20, "starting address"=u16 0, "Modbus master in"=w344) -> ("error out"=w343:errorcluster, "register values"=w356:u16[], "Modbus master out"=w367:refnum<class "Modbus Master.lvclass">)  [unwired: 6 in]
        "Values Read3" <- w356
        n131 = Merge Errors(w343, w341) -> (w342:errorcluster)
        n132 = Index Array(array=w356, index=0) -> (element=w355:u16)
        "PositionLow3" <- w355
        n133 = Index Array(array=w356, index=1) -> (element=w354:u16)
        "PositionHigh3" <- w354
        n134 = Index Array(array=w356, index=4) -> (element=w350:u16)
        n135 = Index Array(array=w356, index=7) -> (element=w359:u16)
        n136 = Index Array(array=w356, index=3) -> (element=w352:u16)
        n137 = To Word Integer(number=w352) -> (16bit integer=w351:i16)
        n138 = To Word Integer(number=w350) -> (16bit integer=w349:i16)
        "SpeedRPM3" <- w349
        n139 = Divide(x=w359, y=100.0) -> (x/y=→"Motor Current3":dbl)
        n140 = Divide(x=w351, y=1000.0) -> (x/y=→"SpeedRPS3":dbl)
        n141 = Join Numbers(hi=w354, lo=w355) -> ((hi.lo)=→"Position Full3":u32)
        n142 = shared-variable "NI-myRIO-1900-03047493\\Network Variables.lvlib\\SpeedMotor3"(w349, error in=w342) -> (error out=w348:errorcluster)
        n143 = case shown="Error" w348 {
          selector: w348 -> [w375 w378]
          tunnel: [w373 w376] -> w370
          tunnel: [w375 w378] -> w372
          tunnel: w367 -> [w374 w377]
          tunnel: [w374 w377] -> w371
          frame No Error {
            w373 = Modbus."Read Slave 4"  # Modbus Enum
          }
          frame Error {
            w376 = Modbus."Read Slave 4"  # Modbus Enum
          }
        }
      }
      frame "Read Slave 4" {
        n144 = call <vilib>:"Set Unit ID.vi"("error in (no error)"=w384, "unit ID"=u8 4, "Modbus master in"=w383) -> ("error out"=w379:errorcluster, "Modbus master out"=w385:refnum<class "Modbus Master.lvclass">)  [unwired: 7 in]
        n145 = call-dynamic "Read Holding Registers.vi"("number of holding registers"=u16 20, "starting address"=u16 0, "Modbus master in"=w385) -> ("error out"=w380:errorcluster, "register values"=w394:u16[], "Modbus master out"=w405:refnum<class "Modbus Master.lvclass">)  [unwired: 6 in]
        "Values Read4" <- w394
        n146 = Merge Errors(w380, w379) -> (w381:errorcluster)
        n147 = Index Array(array=w394, index=0) -> (element=w393:u16)
        "PositionLow4" <- w393
        n148 = Index Array(array=w394, index=1) -> (element=w392:u16)
        "PositionHigh4" <- w392
        n149 = Index Array(array=w394, index=4) -> (element=w388:u16)
        n150 = Index Array(array=w394, index=7) -> (element=w397:u16)
        n151 = Index Array(array=w394, index=3) -> (element=w390:u16)
        n152 = To Word Integer(number=w390) -> (16bit integer=w389:i16)
        n153 = To Word Integer(number=w388) -> (16bit integer=w387:i16)
        "SpeedRPM4" <- w387
        n154 = Divide(x=w397, y=100.0) -> (x/y=→"Motor Current4":dbl)
        n155 = Divide(x=w389, y=1000.0) -> (x/y=→"SpeedRPS4":dbl)
        n156 = Join Numbers(hi=w392, lo=w393) -> ((hi.lo)=→"Position Full4":u32)
        n157 = shared-variable "NI-myRIO-1900-03047493\\Network Variables.lvlib\\SpeedMotor4"(w387, error in=w381) -> (error out=w386:errorcluster)
        n158 = case shown="Error" w386 {
          selector: w386 -> [w413 w416]
          tunnel: [w411 w414] -> w408
          tunnel: [w413 w416] -> w410
          tunnel: w405 -> [w412 w415]
          tunnel: [w412 w415] -> w409
          frame No Error {
            w411 = Modbus."Read Slave 5"  # Modbus Enum
          }
          frame Error {
            w414 = Modbus."Read Slave 5"  # Modbus Enum
          }
        }
      }
      frame "Read Slave 5" {
        n159 = call <vilib>:"Set Unit ID.vi"("error in (no error)"=w452, "unit ID"=u8 5, "Modbus master in"=w451) -> ("error out"=w447:errorcluster, "Modbus master out"=w453:refnum<class "Modbus Master.lvclass">)  [unwired: 7 in]
        n160 = call-dynamic "Read Holding Registers.vi"("number of holding registers"=u16 20, "starting address"=u16 0, "Modbus master in"=w453) -> ("error out"=w448:errorcluster, "register values"=w420:u16[], "Modbus master out"=w455:refnum<class "Modbus Master.lvclass">)  [unwired: 6 in]
        "Values Read5" <- w420
        n161 = Merge Errors(w448, w447) -> (w449:errorcluster)
        n162 = Index Array(array=w420, index=12) -> (element=w419:u16)
        n163 = Index Array(array=w420, index=3) -> (element=w422:u16)
        n164 = Index Array(array=w420, index=1) -> (element=w439:u16)
        n165 = Index Array(array=w420, index=0) -> (element=w440:u16)
        n166 = To Word Integer(number=w440) -> (16bit integer=w428:i16)
        n167 = To Word Integer(number=w439) -> (16bit integer=w426:i16)
        n168 = To Word Integer(number=w419) -> (16bit integer=w418:i16)
        n169 = To Double Precision Float(number=w426) -> (double precision float=w425:dbl)
        n170 = To Double Precision Float(number=w428) -> (double precision float=w427:dbl)
        n171 = To Double Precision Float(number=w418) -> (double precision float=→"PSoC PID Value":dbl)
        n172 = To Double Precision Float(number=w422) -> (double precision float=w424:dbl)
        n173 = Divide(x=w427, y=10.0) -> (x/y=w437:dbl)
        "X" <- w437
        n174 = Divide(x=w425, y=10.0) -> (x/y=w435:dbl)
        "Y" <- w435
        n175 = Divide(x=w424, y=10.0) -> (x/y=→"PSoC Heading":dbl)
        n176 = Add(x=w437, y=-34.0) -> (x+y=w433:dbl)
        n177 = Add(x=w435, y=502.0) -> (x+y=w429:dbl)
        n178 = Inverse Tangent (2 Input)(1:w433, 2:w429) -> (0:w431:dbl)
        n179 = Less Than 0?(x=w431) -> (x < 0?=w432:bool)
        n180 = case shown="True" w432 {
          tunnel: w431 -> [w461 w466]
          tunnel: [w461 w465] -> w430
          frame False {
          }
          frame True {
            n181 = Multiply(x=3.141592653589793, y=2.0) -> (x*y=w462:dbl)
            n182 = Add(x=w466, y=w462) -> (x+y=w465:dbl)
          }
        }
        n183 = expression code="(x/pi)*180.0" "radians to degrees"(w430) -> (w423:dbl)
        "LabVIEW Heading" <- w423
        n184 = shared-variable "NI-myRIO-1900-03047493\\Network Variables.lvlib\\CompassHeading"(w423, error in=w449) -> (error out=w454:errorcluster)
        n185 = case shown="Error" w454 {
          selector: w454 -> [w469 w472]
          tunnel: [w467 w470] -> w458
          tunnel: [w469 w472] -> w460
          tunnel: w455 -> [w468 w471]
          tunnel: [w468 w471] -> w459
          frame No Error {
            w467 = Modbus."Write Slave 1"  # Modbus Enum
          }
          frame Error {
            w470 = Modbus."Close Master"  # Modbus Enum
          }
        }
      }
      frame "Close Master" {
        w473 = Modbus."Create Master"  # Modbus Enum
        n186 = call-dynamic "Close.vi"("error in (no error)"=w476, "Modbus master in"=w477) -> ()  [unwired: 9 in, 1 out]
      }
      frame "TestReadCoils4" {
        w482 = u16 0  # starting address
        n187 = call-dynamic "Read Coils.vi"("error in (no error)"=w483, "number of coils"="Read Count 2", "starting address"=w482, "Modbus master in"=w484) -> ("error out"=w479:errorcluster, "coil values"=→"Coil Values Read":bool[], "Modbus master out"=w481:refnum<class "Modbus Master.lvclass">)  [unwired: 5 in]
        n188 = case shown="No Error" w479 {
          selector: w479 -> [w490 w493]
          tunnel: [w488 w491] -> w478
          tunnel: [w490 w493] -> w487
          tunnel: w481 -> [w489 w492]
          tunnel: [w489 w492] -> w480
          frame No Error {
            w488 = Modbus."TestWriteCoils4"  # Modbus Enum
          }
          frame Error {
            w491 = Modbus."TestReadCoils4"  # Modbus Enum
          }
        }
      }
      frame "TestWriteCoils4" {
        n189 = call-dynamic "Write Multiple Coils.vi"("error in (no error)"=w499, "coil values"="Coil Values to Write", "starting address"=u16 0, "Modbus master in"=w500) -> ("error out"=w498:errorcluster, "Modbus master out"=w497:refnum<class "Modbus Master.lvclass">)  [unwired: 6 in]
        n190 = case shown="No Error" w498 {
          selector: w498 -> [w504 w507]
          tunnel: w497 -> [w505 w508]
          tunnel: [w503 w506] -> w496
          tunnel: [w505 w508] -> w495
          tunnel: [w504 w507] -> w494
          frame No Error {
            w503 = Modbus."TestReadCoils4"  # Modbus Enum
          }
          frame Error {
            w506 = Modbus."Close Master"  # Modbus Enum
          }
        }
      }
    }
    n191 = call "RT Error HandlerSam.vi"("Ignore Errors"=w15, "Critical Errors"=w14, "queue in"=w13) -> ()  [unwired: 8 in, 1 out]
  }
  n192 = call-dynamic "Close.vi"("error in (no error)"=w3, "Modbus master in"=w4) -> ()  [unwired: 9 in, 1 out]
